vi "Classify Token.vi"(8 "Error In":errorcluster, 11 "Parser In":refnum<class "Parser.lvclass">) -> (0 "Error Out":errorcluster, 2 "Class":T1, 3 "Parser Out":refnum<class "Parser.lvclass">)   [LabVIEW 2017, in "Mustache.lvlib" / "Parser.lvclass"]
uses:
  Parser.lvclass
  Token Class.ctl
  Parser.lvclass/Parser.ctl
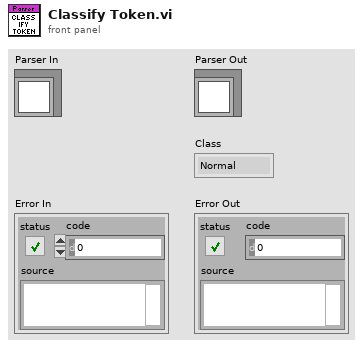
[diagram p1: front panel]
types:
  T1 = typedef "Mustache.lvlib/Parser.lvclass/Token Class.ctl" = enum16{"Normal", "Stand Alone", "Whitespace"}
  T2 = typedef "Mustache.lvlib/Parser.lvclass/Token.ctl" = cluster{"Type":T3, "Data":variant}
  T3 = typedef "Mustache.lvlib/Parser.lvclass/Token Types.ctl" = enum16{"Text", "Escaped Tag", "Unescaped Tag", "Section", "Incomplete Section", "Partial"}
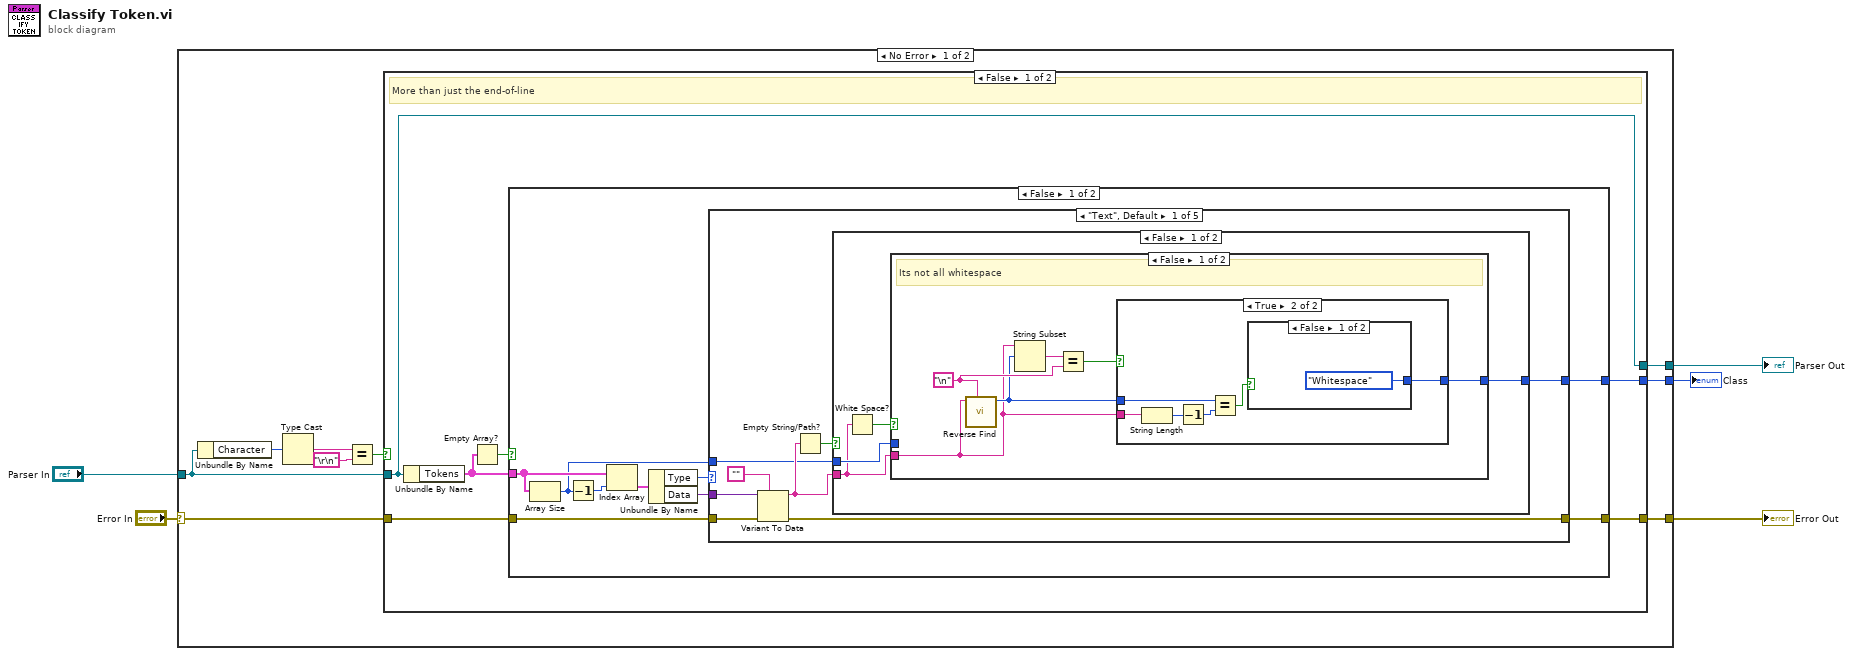
[diagram p0: block diagram]
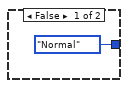
[diagram p2: hidden frame]
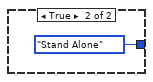
[diagram p3: hidden frame]
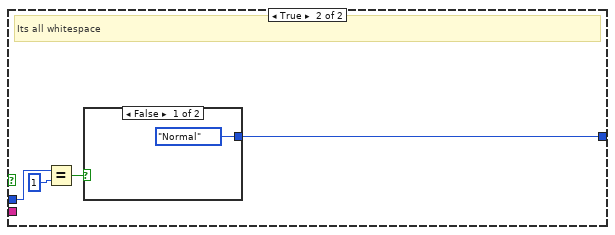
[diagram p4: hidden frame]
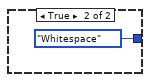
[diagram p5: hidden frame]
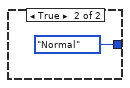
[diagram p6: hidden frame]
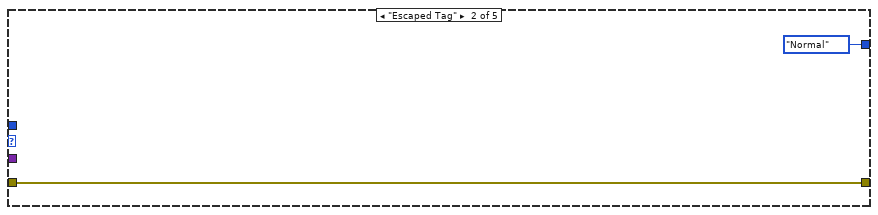
[diagram p7: hidden frame]
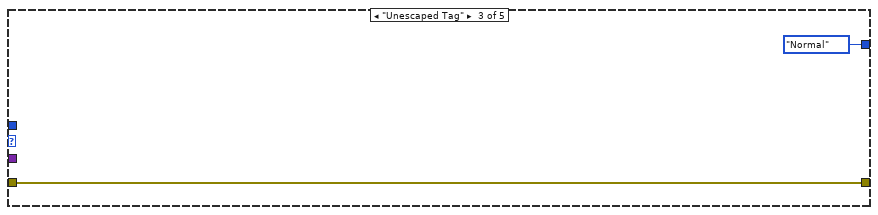
[diagram p8: hidden frame]
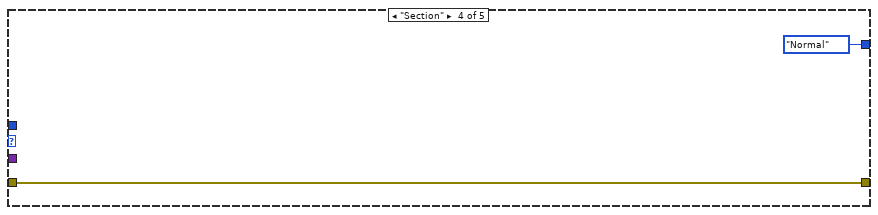
[diagram p9: hidden frame]
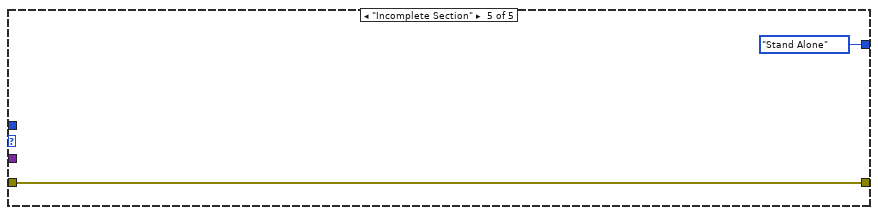
[diagram p10: hidden frame]
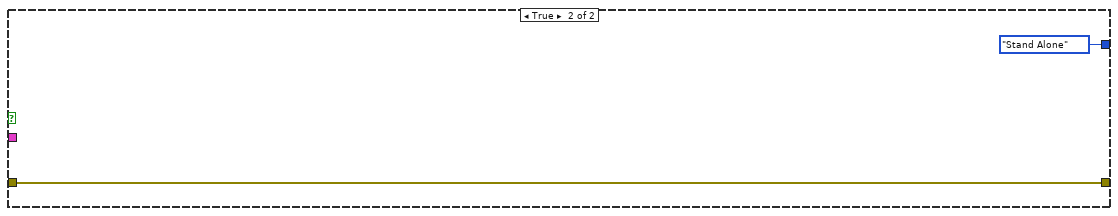
[diagram p11: hidden frame]
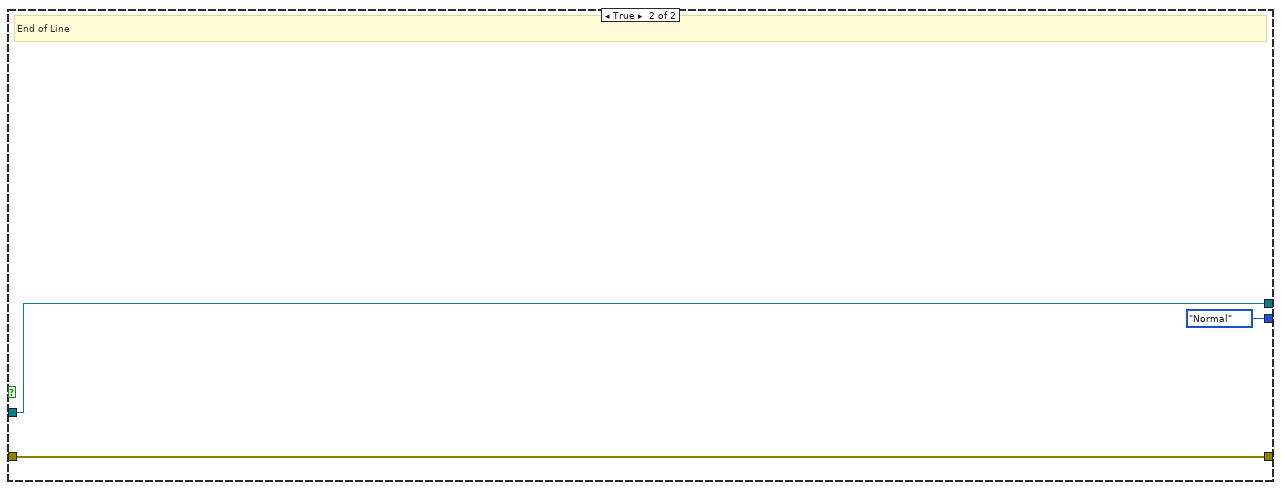
[diagram p12: hidden frame]
diagram:
  n1 = case shown="No Error" "Error In" {
    selector: "Error In" -> [w8 w78]
    tunnel: "Parser In" -> [w9 w77]
    tunnel: [w7 w78] -> w3
    tunnel: [w6 w77] -> w2
    tunnel: [w10 _] -> w1
    frame No Error {
      n2 = Unbundle By Name(w9) -> ("Character"=w14:u8)
      n3 = Type Cast(x=w14) -> (*(type *) &x=w13:string)  [unwired: 1 in]
      n4 = Equal?(x=w13, y="\r\n") -> (x = y?=w11:bool)
      n5 = case shown="False" w11 {
        tunnel: [w19 Token_Class."Normal" ("Class")] -> w10
        tunnel: w9 -> [w15 w74]
        tunnel: w8 -> [w17 w75]
        tunnel: [w16 w75] -> w7
        tunnel: [w15 w74] -> w6
        frame False {
          # "More than just the end-of-line"
          n6 = Unbundle By Name(w15) -> ("Tokens"=w18:T2[])
          n7 = Empty Array?(array=w18) -> (empty?=w20:bool)
          n8 = case shown="False" w20 {
            tunnel: [w25 Token_Class."Stand Alone" ("Class")] -> w19
            tunnel: w18 -> [w29 _]
            tunnel: w17 -> [w23 w72]
            tunnel: [w22 w72] -> w16
            frame False {
              n9 = Array Size(array=w29) -> (size(s)=w21:i32)
              n10 = Decrement(x=w21) -> (x-1=w28:i32)
              n11 = Index Array(array=w29, index=w28) -> (element=w27:T2)
              n12 = Unbundle By Name(w27) -> ("Type"=w26:T3, "Data"=w24:variant)
              n13 = case shown="\"Text\", Default" w26 {
                tunnel: [w32 Token_Class."Normal" ("Class") Token_Class."Normal" ("Class") Token_Class."Normal" ("Class") Token_Class."Stand Alone" ("Class")] -> w25
                tunnel: w24 -> [w37 _ _ _ _]
                tunnel: w23 -> [w35 w64 w67 w69 w70]
                tunnel: [w34 w64 w67 w69 w70] -> w22
                tunnel: w21 -> [w30 _ _ _ _]
                frame "Text", Default {
                  n14 = Variant To Data(error in=w35, type="", Variant=w37) -> (data=w31:string, error out=w34:errorcluster)
                  n15 = Empty String/Path?(string/path=w31) -> (empty?=w33:bool)
                  n16 = case shown="False" w33 {
                    tunnel: [w39 Token_Class."Normal" ("Class")] -> w32
                    tunnel: w31 -> [w38 _]
                    tunnel: w30 -> [w40 _]
                    frame False {
                      n17 = White Space?(1:w38) -> (0:w41:bool)
                      n18 = case shown="False" w41 {
                        tunnel: w40 -> [_ w60]
                        tunnel: [w44 w57] -> w39
                        tunnel: w38 -> [w42 _]
                        frame False {
                          w46 = "\n"
                          # "Its not all whitespace"
                          n19 = call "Reverse Find.vi"("Character"=w46, "String"=w42) -> ("Position"=w43:i32)  [unwired: 9 in]
                          n20 = String Subset(string=w42, offset (0)=w43) -> (substring=w47:string)  [unwired: 1 in]
                          n21 = Equal?(x=w47, y=w46) -> (x = y?=w45:bool)
                          n22 = case shown="True" w45 {
                            tunnel: [Token_Class."Normal" ("Class") w49] -> w44
                            tunnel: w43 -> [_ w54]
                            tunnel: w42 -> [_ w53]
                            frame False {
                            }
                            frame True {
                              n23 = String Length(string=w53) -> (length=w52:i32)
                              n24 = Decrement(x=w52) -> (x-1=w51:i32)
                              n25 = Equal?(x=w54, y=w51) -> (x = y?=w50:bool)
                              n26 = case shown="False" w50 {
                                tunnel: [Token_Class."Whitespace" ("Class") Token_Class."Stand Alone" ("Class")] -> w49
                                frame False {
                                }
                                frame True {
                                }
                              }
                            }
                          }
                        }
                        frame True {
                          # "Its all whitespace"
                          n27 = Equal?(x=w60, y=1) -> (x = y?=w58:bool)
                          n28 = case shown="False" w58 {
                            tunnel: [Token_Class."Normal" ("Class") Token_Class."Whitespace" ("Class")] -> w57
                            frame False {
                            }
                            frame True {
                            }
                          }
                        }
                      }
                    }
                    frame True {
                    }
                  }
                }
                frame "Escaped Tag" {
                }
                frame "Unescaped Tag" {
                }
                frame "Section" {
                }
                frame "Incomplete Section" {
                }
              }
            }
            frame True {
            }
          }
        }
        frame True {
          # "End of Line"
        }
      }
    }
    frame Error {
    }
  }
  "Error Out" <- w3
  "Parser Out" <- w2
  "Class" <- w1
